vi "RemoteControl.SendMessageToProcess.vi"(8 "error in (no error)":errorcluster, 10 "Message":T1={"Command"="", "Data"=variant(string ""), "ID"="", "error"={"status"=FALSE, "code"=0, "source"=""}}, 11 "RemoteControl":refnum<class "RemoteControl.lvclass">) -> (0 "error out":errorcluster, 3 "RemoteControl out":refnum<class "RemoteControl.lvclass">)   [LabVIEW 2019, in "RemoteControl.lvlib" / "RemoteControl.lvclass"]
doc: "---------------------------------------------------------------\nJKI State Machine Objects™\nhttp://jki.net/state-machine-objects/\nCopyright (C) 2005-2015, JKI <info@jki.net>\nALL RIGHTS RESERVEDJKI State Machine Objects (SMO) 1.0.0.4\nJKI - JKI\nCopyright (c) 2015, JKI"
uses:
  RemoteControl.lvclass
  Typedefs/Message--Cluster.ctl
  RemoteControl.lvclass/RemoteControl.ctl
  Typedefs/PrivateEvents--RemoteControl.SendMessageToProcess.ctl
panel:
  # "For instructions on how to use the JKI State Machine Objects, examples and video tutorials, visit:\nhttp://jki.net/state-machine-objects/\n\nJKI State Machine Objects™\nhttp://jki.net/state-machine-objects/\nCopyright (C) 2005-2015, JKI <info@jki.net>\nALL RIGHTS RESERVED"
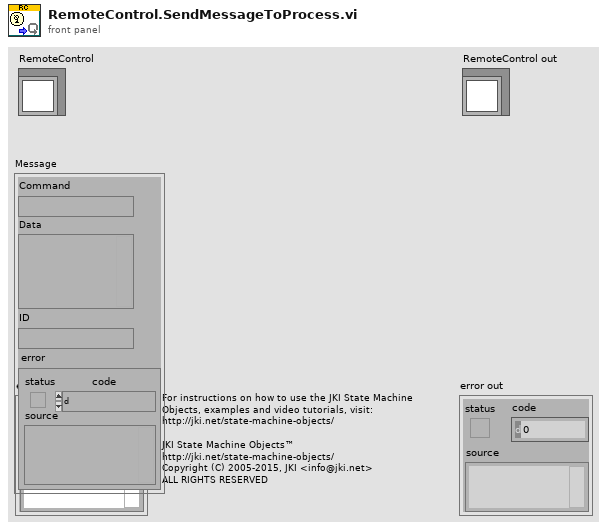
[diagram p1: front panel]
types:
  T1 = typedef "RemoteControl.lvlib/RemoteControl.lvclass/Message--Cluster.ctl" = cluster{"Command":string, "Data":variant, "ID":string, "error":errorcluster}
  T2 = typedef "RemoteControl.lvlib/RemoteControl.lvclass/PrivateEvents--RemoteControl.SendMessageToProcess.ctl" = cluster{"Message":T1}
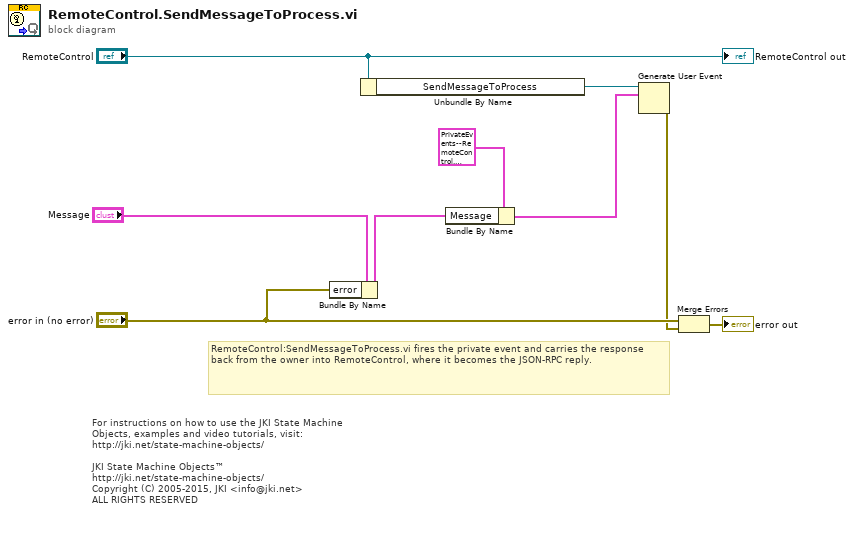
[diagram p0: block diagram]
diagram:
  # "RemoteControl:SendMessageToProcess.vi fires the private event and carries the response back from the owner into RemoteControl, where it becomes the JSON-RPC reply."
  # "For instructions on how to use the JKI State Machine Objects, examples and video tutorials, visit:\nhttp://jki.net/state-machine-objects/\n\nJKI State Machine Objects™\nhttp://jki.net/state-machine-objects/\nCopyright (C) 2005-2015, JKI <info@jki.net>\nALL RIGHTS RESERVED"
  n1 = Bundle By Name(cluster="Message", "error"="error in (no error)") -> (w4:T1)
  n2 = Unbundle By Name("RemoteControl") -> ("SendMessageToProcess"=w6:refnum<user-event>)
  n3 = Bundle By Name(cluster=T2 {"Message"={"Command"="", "Data"=variant(string ""), "ID"="", "error"={"status"=FALSE, "code"=0, "source"=""}}} ("SendMessageToProcess"), "Message"=w4) -> (w7:T2)
  n4 = Generate User Event(user event=w6, event data cluster=w7) -> (error out=w2:errorcluster)  [unwired: 2 in, 1 out]
  n5 = Merge Errors("error in (no error)", w2) -> (→"error out":errorcluster)
  "RemoteControl out" <- "RemoteControl"
